vi "InitializeLog.vi"() -> (3 "Byte Stream File out":refnum<file>)   [LabVIEW 2016]
panel:
  in  "Format":string="==============================================================================================================================\nTIME\tL1_cmd\tL2_cmd\tL3_cmd\tL4_cmd\tL1_out\tL2_out\tL3_out\tL4_out\tStageX\tStageY\tStageZ\tI_out\tA_out\tCurrentSate\tIrisCenter_X\tIrisCener_Y\tIrisScaling_X\tIrisScaling_Y\tAN_NoFly\tAN_Cruising\tIrisCenter_Z\tPO_Cruising\tPO_NoFly\n=============================================================================================================================="
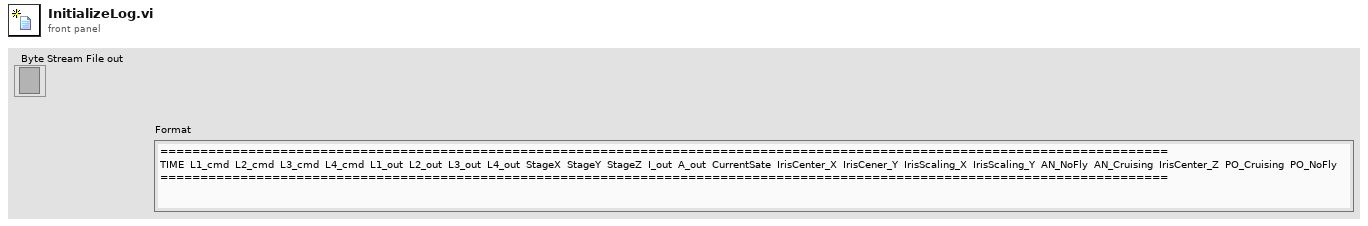
[diagram p1: front panel]
types:
  T1 = enum16{"open", "replace", "create", "open or create", "replace or create", "replace or create with confirmation"}
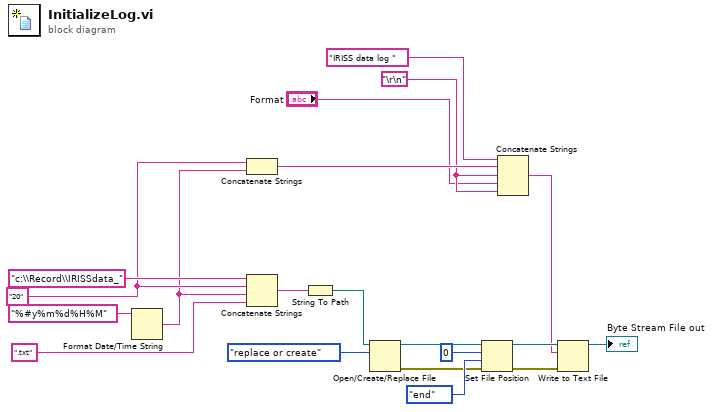
[diagram p0: block diagram]
diagram:
  w2 = "\r\n"
  w5 = "20" ("string")
  n1 = Format Date/Time String(time format string (%c)="%#y%m%d%H%M" ("string")) -> (date/time string=w4:string)  [unwired: 2 in]
  n2 = Concatenate Strings(w5, w4) -> (w3:string)
  n3 = Concatenate Strings("c:\\Record\\IRISSdata_" ("string"), w5, w4, ".txt" ("string")) -> (w6:string)
  n4 = String To Path(string=w6) -> (path=w17:path)
  n5 = Open/Create/Replace File(file path (use dialog)=w17, operation (0:open)=T1."replace or create") -> (refnum out=w15:refnum<file>, error out=w10:errorcluster)  [unwired: 4 in, 1 out]
  n6 = Set File Position(offset (in bytes) (0)=i64 0, refnum=w15, from (0:start)=enum16{"start", "end", "current"}."end", error in=w10) -> (refnum out=w12:refnum<file>, error out=w9:errorcluster)
  n7 = Concatenate Strings("IRISS data log " ("string"), w3, w2, "Format", w2) -> (w8:string)
  n8 = Write to Text File(file (use dialog)=w12, text=w8, error in=w9) -> (refnum out=→"Byte Stream File out":refnum<file>)  [unwired: 1 in, 2 out]
